vi "localUserCheck.vi"(0 "xmlConfigPath":path caption="XML文档路径", 7 "name":string, 9 "psw":string, 11 "error in (no error)":errorcluster caption="错误输入（无错误）") -> (4 "userList":string[](array[string]), 15 "错误输出":errorcluster)   [LabVIEW 2011]
uses:
  D:/gitProjects/HPTS_VNA/Data/xmlFunction.dll
  Data/xmlFunction.dll
  <vilib>/xml/Load XML File.vi
  <vilib>/xml/Close Reference(Node).vi
  <vilib>/xml/NI_XML.lvlib
  C:/Program Files (x86)/National Instruments/LabVIEW 2011/resource/objmgr/DOMUserDefRef.rc
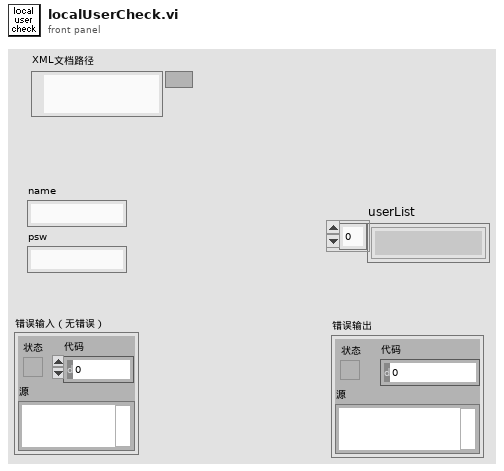
[diagram p1: front panel]
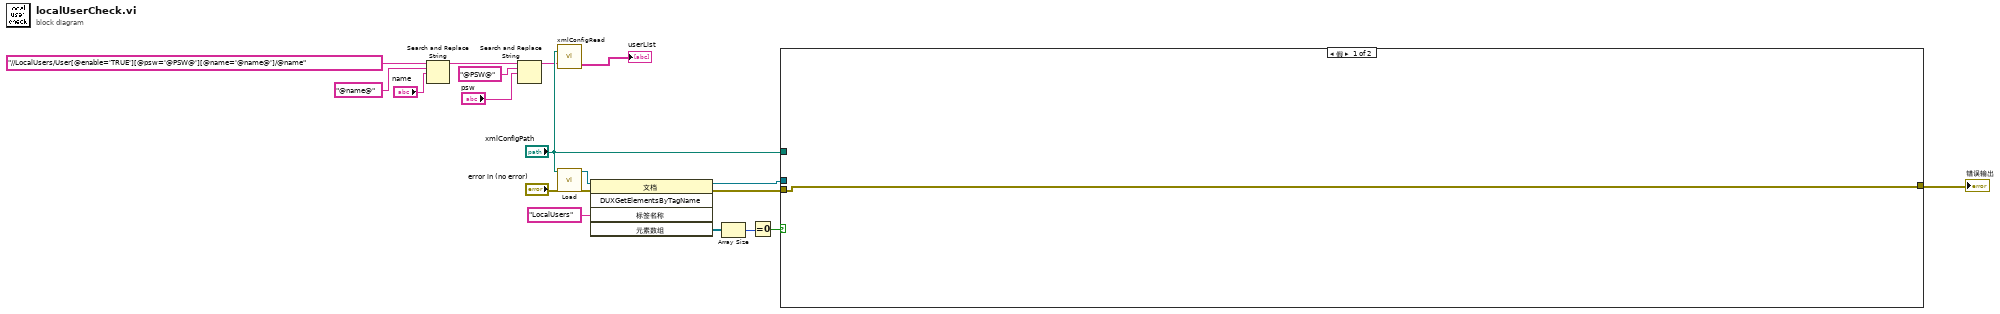
[diagram p0: block diagram]
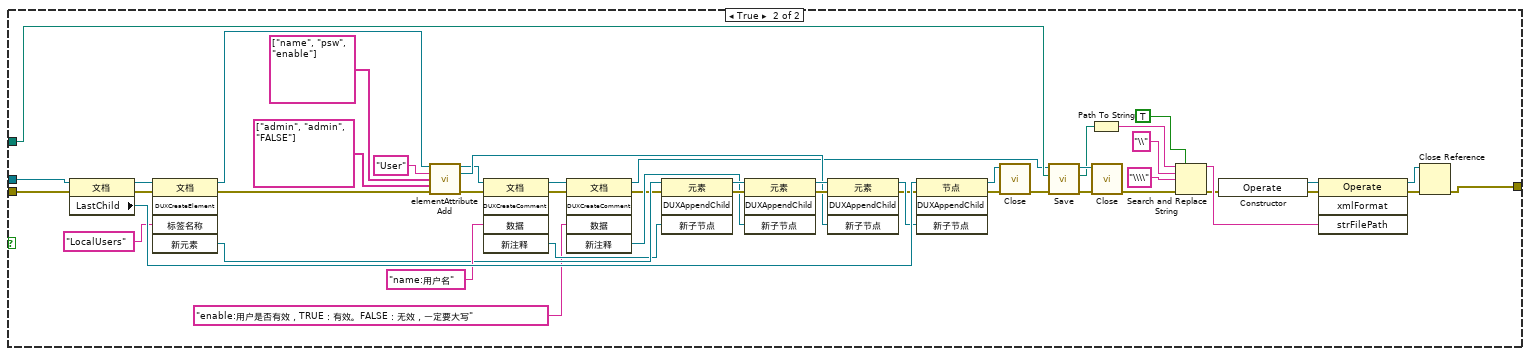
[diagram p2: hidden frame]
diagram:
  n1 = Search and Replace String(input string="//LocalUsers/User[@enable='TRUE'][@psw='@PSW@'][@name='@name@']/@name" ("XPath expression"), search string="@name@" ("搜索字符串"), replace string="name") -> (result string=w5:string)  [unwired: 5 in, 3 out]
  n2 = Search and Replace String(input string=w5, search string="@PSW@" ("搜索字符串"), replace string="psw") -> (result string=w1:string)  [unwired: 5 in, 3 out]
  n3 = call "xmlConfigRead.vi"("path to XML document"="xmlConfigPath", "XPath expression"=w1) -> ("OutParaArray"=→"userList":string[])  [unwired: 2 out]
  n4 = call-poly <vilib>:"Load.vi"("path to XML document"="xmlConfigPath", "error in (no error)"="error in (no error)") -> ("DOM document out"=w18:refnum<k20>, "error out"=w12:errorcluster)  [unwired: 11 in, 1 out]
  n5 = invoke class="文档" method="DUXGetElementsByTagName"(reference=w18, error in=w12, "标签名称"="LocalUsers") -> (reference out=w13:refnum<k20>, error out=w11:errorcluster, "元素数组"=w16:refnum<k20>[])  [unwired: 2 in, 2 out]
  n6 = Array Size(array=w16) -> (size(s)=w15:i32)
  n7 = Equal To 0?(x=w15) -> (x = 0?=w14:bool)
  n8 = case shown="假" w14 {
    tunnel: "xmlConfigPath" -> [_ w68]
    tunnel: w11 -> [w20 w43]
    tunnel: w13 -> [_ w33]
    tunnel: [w20 w21] -> w2
    frame False {
    }
    frame True {
      n9 = property class="文档"(reference=w33, error in=w43) -> (reference out=w66:refnum<k20>, error out=w64:errorcluster, "LastChild"=w67:refnum<k20>)
      n10 = invoke class="文档" method="DUXCreateElement"(reference=w66, error in=w64, "标签名称"="LocalUsers") -> (reference out=w39:refnum<k20>, error out=w36:errorcluster, "新元素"=w53:refnum<k20>)  [unwired: 2 in, 2 out]
      n11 = call "elementAttributeAdd.vi"("DOM document in"=w39, "elementName"="User" ("标签名称"), "property"=string[] ["name", "psw", "enable"], "value"=string[] ["admin", "admin", "FALSE"], "错误输入（无错误）"=w36) -> ("DOM document out"=w25:refnum<k20>, "element"=w34:refnum<k20>, "错误输出"=w24:errorcluster)  [unwired: 8 in]
      n12 = invoke class="文档" method="DUXCreateComment"(reference=w25, error in=w24, "数据"="name:用户名") -> (reference out=w48:refnum<k20>, error out=w45:errorcluster, "新注释"=w52:refnum<k20>)  [unwired: 2 in, 2 out]
      n13 = invoke class="文档" method="DUXCreateComment"(reference=w48, error in=w45, "数据"="enable:用户是否有效，TRUE：有效。FALSE：无效，一定要大写") -> (reference out=w26:refnum<k20>, error out=w44:errorcluster, "新注释"=w46:refnum<k20>)  [unwired: 2 in, 2 out]
      n14 = invoke class="元素" method="DUXAppendChild"(reference=w53, error in=w44, "新子节点"=w52) -> (reference out=w51:refnum<k20>, error out=w49:errorcluster)  [unwired: 1 in, 2 out]
      n15 = invoke class="元素" method="DUXAppendChild"(reference=w51, error in=w49, "新子节点"=w46) -> (reference out=w50:refnum<k20>, error out=w35:errorcluster)  [unwired: 1 in, 2 out]
      n16 = invoke class="元素" method="DUXAppendChild"(reference=w50, error in=w35, "新子节点"=w34) -> (reference out=w23:refnum<k20>, error out=w22:errorcluster)  [unwired: 1 in, 2 out]
      n17 = invoke class="节点" method="DUXAppendChild"(reference=w67, error in=w22, "新子节点"=w23) -> (reference out=w54:refnum<k20>, error out=w32:errorcluster)  [unwired: 1 in, 2 out]
      n18 = call-poly <vilib>:"Close.vi"("error in (no error)"=w32, "node"=w54) -> ("error out"=w31:errorcluster)  [unwired: 7 out]
      n19 = call <vilib>:"Save.vi"("error in (no error)"=w31, "XML file path"=w68, "DOM document in"=w26) -> ("error out"=w29:errorcluster, "XML file path out"=w27:path, "DOM document out"=w30:refnum<k20>)  [unwired: 6 in]
      n20 = Path To String(path=w27) -> (string=w63:string)
      n21 = call-poly <vilib>:"Close.vi"("error in (no error)"=w29, "node"=w30) -> ("error out"=w28:errorcluster)  [unwired: 7 in]
      n22 = Search and Replace String(replace all?=TRUE ("替换全部？(F)"), input string=w63, search string="\\" ("搜索字符串"), replace string="\\\\" ("替换字符串(\"\")"), error in=w28) -> (result string=w58:string, error out=w56:errorcluster)  [unwired: 3 in, 2 out]
      n23 = constructor class="Operate"(error in=w56) -> (reference out=w59:refnum<k24>, error out=w57:errorcluster)  [unwired: 2 in, 1 out]
      n24 = invoke class="Operate" method="xmlFormat"(reference=w59, error in=w57, "strFilePath"=w58) -> (reference out=w42:refnum<k24>, error out=w41:errorcluster)  [unwired: 1 in, 2 out]
      n25 = Close Reference(reference=w42, error in (no error)=w41) -> (error out=w21:errorcluster)
    }
  }
  "错误输出" <- w2
